vi "usb_show_video.vi"() -> ()   [LabVIEW 2015]
uses:
  <vilib>/userdefined/High Color/IMAQdx.ctl
  <vilib>/vision/driver/NI_Vision_Acquisition_Software.lvlib
  <resource>/objmgr/imaqdx.rc
panel:
  out "error out":errorcluster
  out "PixelFormat":u32
  out "Image Width":u32
  out "Image Height":u32
  out "Image":T1(plugin-control)
  in  "stop":bool
  in  "Session In":T2
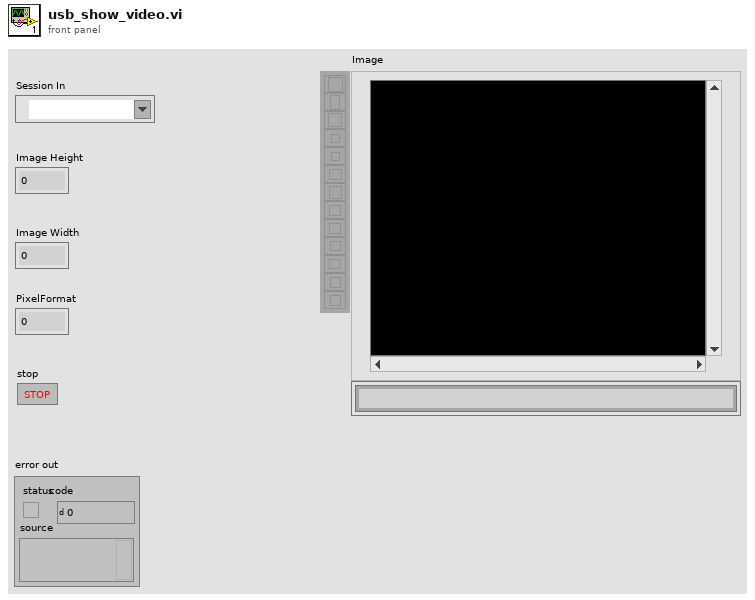
[diagram p1: front panel]
types:
  T1 = typedef "IMAQ Image.ctl" = refnum<image>
  T2 = typedef "IMAQdx.ctl" = refnum<k21>
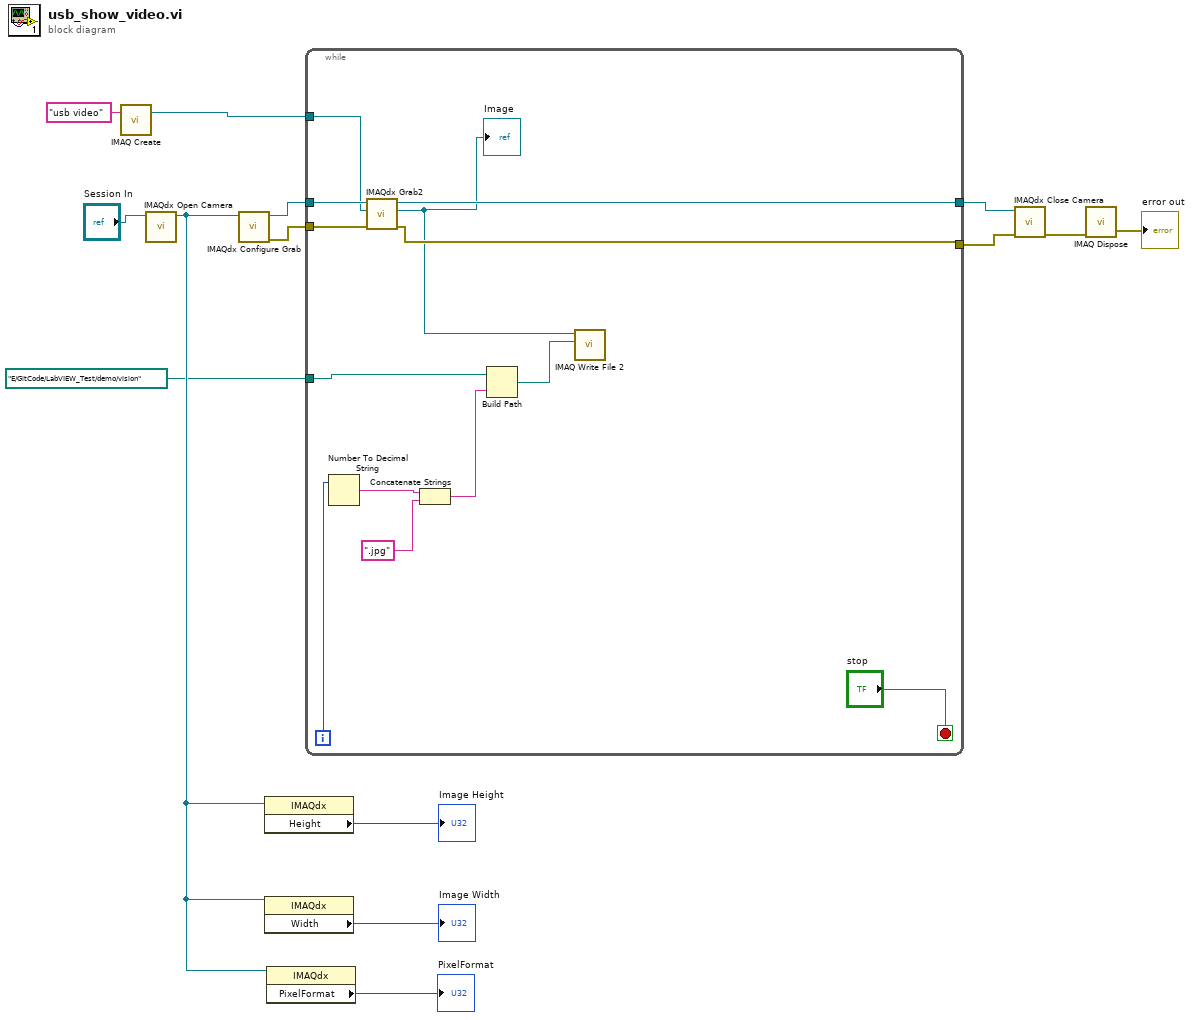
[diagram p0: block diagram]
diagram:
  n1 = call "IMAQ Create"("Image Name"="usb video") -> ("New Image"=w10:T1)  [unwired: 4 in, 1 out]
  n2 = call <vilib>:"IMAQdx Open Camera.vi"("Session In"="Session In") -> ("Session Out"=w4:T2)  [unwired: 9 in, 1 out]
  n3 = call <vilib>:"IMAQdx Configure Grab.vi"("Session In"=w4) -> ("error out"=w12:errorcluster, "Session Out"=w13:T2)  [unwired: 9 in]
  n4 = property class="IMAQdx"(reference=w4) -> ("Height"=→"Image Height":u32)  [unwired: 1 in, 2 out]
  n5 = property class="IMAQdx"(reference=w4) -> ("Width"=→"Image Width":u32)  [unwired: 1 in, 2 out]
  n6 = property class="IMAQdx"(reference=w4) -> ("PixelFormat"=→"PixelFormat":u32)  [unwired: 1 in, 2 out]
  n7 = while {
    tunnel: w13 -> [w27]
    tunnel: w12 -> [w26]
    tunnel: w10 -> [w25]
    tunnel: [w23] -> w9
    tunnel: [w22] -> w8
    tunnel: path "E:/GitCode/LabVIEW_Test/demo/vision" ("base path") -> [w20]
    i -> [w17]
    stop <- "stop" stop-if-true
    n8 = Number To Decimal String(number=w17) -> (decimal integer string=w16:string)  [unwired: 1 in]
    n9 = call <vilib>:"IMAQdx Grab2.vi"("error in"=w26, "Image In"=w25, "Session In"=w27) -> ("error out"=w22:errorcluster, "Image Out"=w21:T1, "Session Out"=w23:T2)  [unwired: 5 in, 1 out]
    "Image" <- w21
    n10 = Concatenate Strings(w16, ".jpg" ("string")) -> (w15:string)
    n11 = Build Path(base path=w20, name or relative path=w15) -> (appended path=w18:path)
    n12 = call-poly "IMAQ Write File 2"("File Path"=w18, "Image"=w21) -> ()  [unwired: 8 in, 2 out]
  }
  n13 = call <vilib>:"IMAQdx Close Camera.vi"("error in"=w8, "Session In"=w9) -> ("error out"=w3:errorcluster)  [unwired: 9 in]
  n14 = call "IMAQ Dispose"("error in (no error)"=w3) -> ("error out"=→"error out":errorcluster)  [unwired: 5 in]
